vi "GDSLvClass_GetClassInfo.vi"(0 "Class Refnum In":refnum<vi>, 5 "error in (no error)":errorcluster) -> (14 "Class Refnum Out":refnum<vi>, 15 "ClassCtl-file":string, 17 "ClassMemberPath":path, 19 "error out":errorcluster)   [LabVIEW 2012]
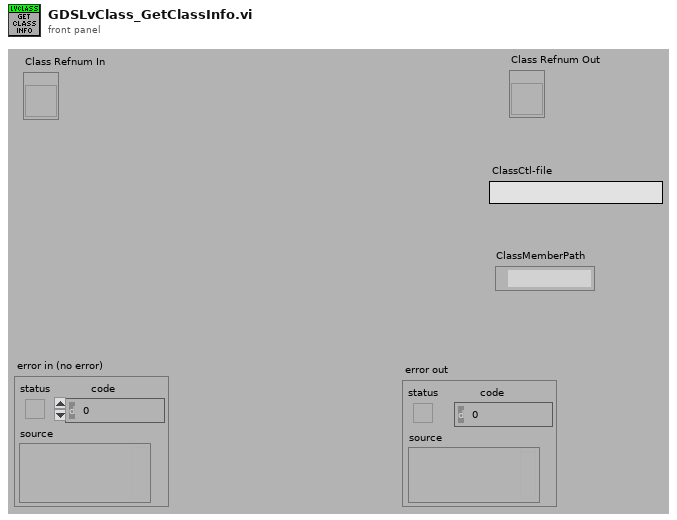
[diagram p1: front panel]
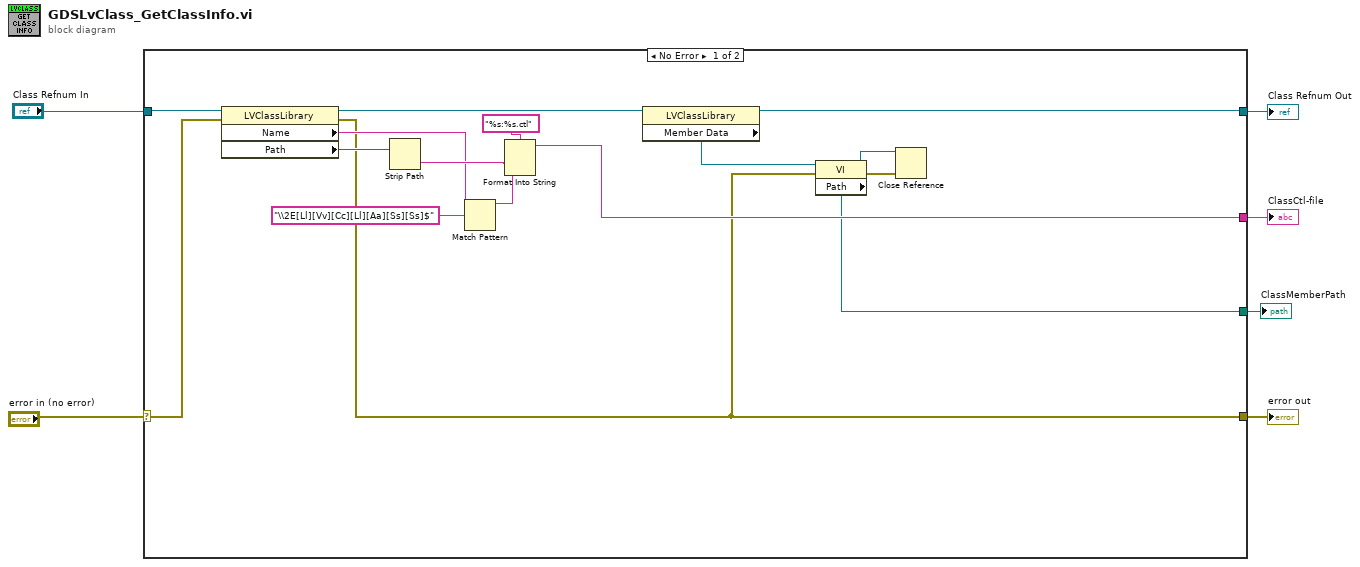
[diagram p0: block diagram]
diagram:
  n1 = case shown="No Error" "error in (no error)" {
    selector: "error in (no error)" -> [w21 w24]
    tunnel: [w10 w24] -> w5
    tunnel: "Class Refnum In" -> [w22 w23]
    tunnel: [w12 w23] -> w3
    tunnel: [w17 _] -> w2
    tunnel: [w9 _] -> w1
    frame No Error {
      n2 = property class="LVClassLibrary"(reference=w22, error in=w21) -> (reference out=w13:refnum<vi>, error out=w10:errorcluster, "Name"=w15:string, "Path"=w20:path)
      n3 = Strip Path(path=w20) -> (name=w19:string)  [unwired: 1 out]
      n4 = Match Pattern(string=w15, regular expression="\\2E[Ll][Vv][Cc][Ll][Aa][Ss][Ss]$") -> (before substring=w14:string)  [unwired: 1 in, 3 out]
      n5 = Format Into String(format string="%s:%s.ctl", w19, w14) -> (resulting string=w17:string)  [unwired: 2 in, 1 out]
      n6 = property class="LVClassLibrary"(reference=w13) -> (reference out=w12:refnum<vi>, "Member Data"=w11:refnum<vi>)  [unwired: 1 in, 1 out]
      n7 = property class="VI"(reference=w11, error in=w10) -> (reference out=w7:refnum<vi>, error out=w8:errorcluster, "Path"=w9:path)
      n8 = Close Reference(reference=w7, error in (no error)=w8) -> ()  [unwired: 1 out]
    }
    frame Error {
    }
  }
  "Class Refnum Out" <- w3
  "error out" <- w5
  "ClassCtl-file" <- w2
  "ClassMemberPath" <- w1
